vi "Joystick_Control.vi"() -> ()   [LabVIEW 2018]
uses:
  TypeDefs/JoystickControls.ctl
panel:
  in  "Joystick control":T1
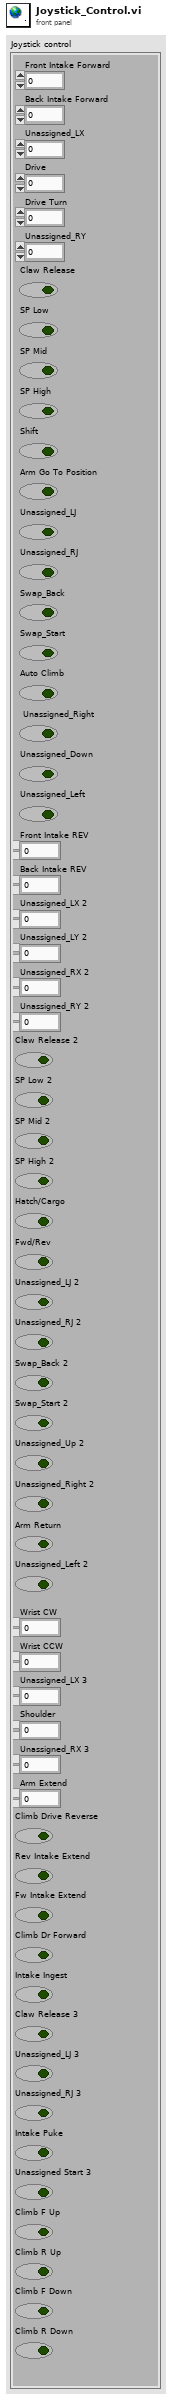
[diagram p1: front panel]
types:
  T1 = typedef "JoystickControls.ctl" = cluster{"Drive":dbl, "Drive Turn ":dbl, "Unassigned_LX":dbl, "Unassigned_RY":dbl, "Claw Release":bool, "Back Intake Forward":dbl, "Front Intake Forward":dbl, "SP Low":bool, "SP Mid":bool, "SP High":bool, "Shift":bool, "Arm Go To Position":bool, "Unassigned_LJ":bool, "Unassigned_RJ":bool, "Swap_Back":bool, "Swap_Start":bool, "Unassigned_LY 2":dbl, "Unassigned_RX 2":dbl, "Unassigned_LX 2":dbl, "Unassigned_RY 2":dbl, "Claw Release 2":bool, "Back Intake REV":dbl, "Front Intake REV":dbl, "SP Low 2":bool, "SP Mid 2":bool, "SP High 2":bool, "Hatch/Cargo":bool, "Fwd/Rev":bool, "Unassigned_LJ 2":bool, "Unassigned_RJ 2":bool, "Swap_Back 2":bool, "Swap_Start 2":bool, "Unassigned_Up 2":bool, "Unassigned_Right 2":bool, "Arm Return":bool, "Unassigned_Left 2":bool, "Auto Climb":bool, " Unassigned_Right":bool, "Unassigned_Down":bool, "Unassigned_Left":bool, "Shoulder":dbl, "Unassigned_RX 3":dbl, "Unassigned_LX 3":dbl, "Arm Extend":dbl, "Climb Drive Reverse":bool, "Wrist CCW":dbl, "Wrist CW":dbl, "Rev Intake Extend":bool, "Fw Intake Extend":bool, "Climb Dr Forward":bool, "Intake Ingest ":bool, "Claw Release 3":bool, "Unassigned_LJ 3":bool, "Unassigned_RJ 3":bool, "Intake Puke":bool, "Unassigned Start 3":bool, "Climb F Up":bool, "Climb R Up":bool, "Climb F Down":bool, "Climb R Down":bool}
diagram:
